vi "GD_GWID7S_info.vi"(8 "error in (no error)":errorcluster, 9 "glue_p2":sgl, 10 "glue_id":string, 11 "DBlink":string="Driver={ODBC Driver 17 for SQL Server};Server=localhost\\SQLEXPRESS;Database=ZDX201;UID=labview;PWD=Dsa@54137926") -> (0 "error out":errorcluster)   [LabVIEW 2019]
uses:
  <vilib>/addons/database/Connection.llb/DB Tools Open Connec (String).vi
  <vilib>/addons/database/NI_Database_API.lvlib
panel:
  out "Command 2":string="WHERE [id]=16"
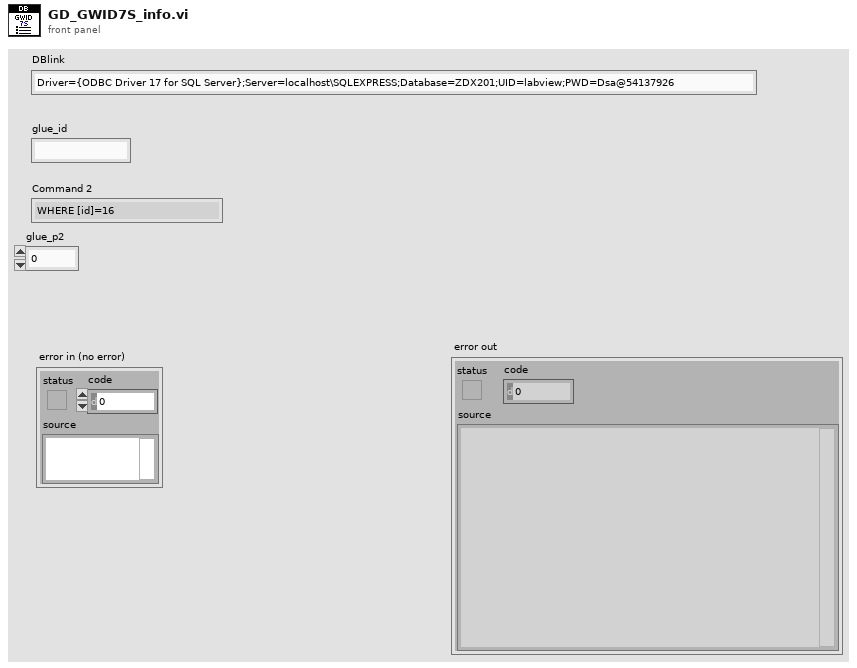
[diagram p1: front panel]
types:
  T1 = cluster{"update_time":timestamp, "time_standby_2":timestamp, "glue_p2":sgl}
  T2 = typedef "NI_Database_API.lvlib/Conn ObjectReference.ctl" = refnum<k1>
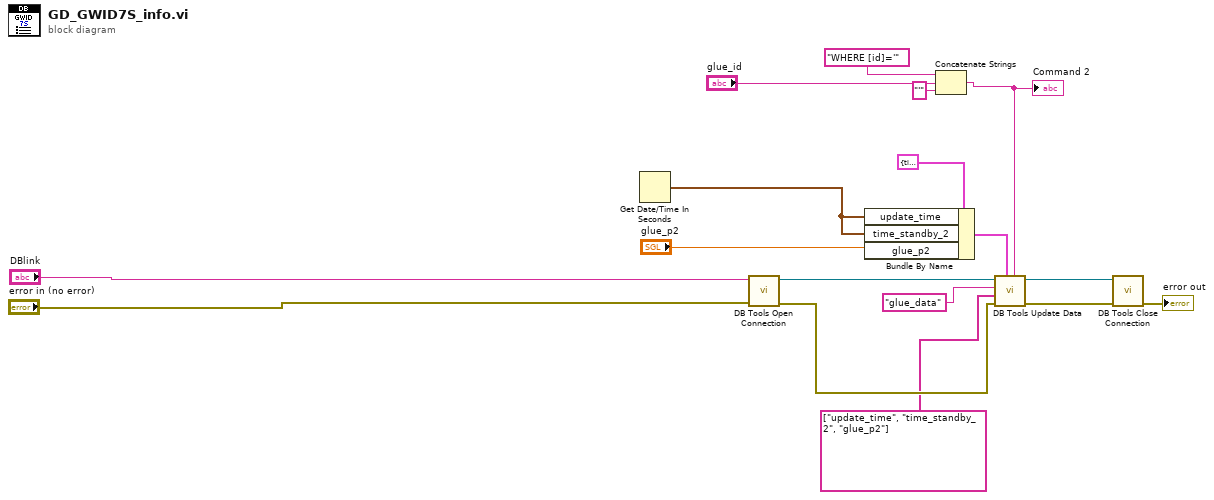
[diagram p0: block diagram]
diagram:
  n1 = Get Date/Time In Seconds() -> (seconds since 1Jan1904=w8:timestamp)
  n2 = call-poly <vilib>:"DB Tools Open Connection.vi"("error in (no error)"="error in (no error)", "connection information"="DBlink") -> ("error out"=w16:errorcluster, "connection reference"=w9:T2)  [unwired: 6 in]
  n3 = Bundle By Name(cluster=T1 {"update_time"=timestamp(0 s since 1904-01-01), "time_standby_2"=timestamp(0 s since 1904-01-01), "glue_p2"=0.0}, "update_time"=w8, "time_standby_2"=w8, "glue_p2"="glue_p2") -> (w10:T1)
  n4 = Concatenate Strings("WHERE [id]='", "glue_id", "'" ("string")) -> (w5:string)
  "Command 2" <- w5
  n5 = call <vilib>:"DB Tools Update Data.vi"("condition"=w5, "data"=w10, "error in (no error)"=w16, "columns"=string[] ["update_time", "time_standby_2", "glue_p2"], "table"="glue_data", "connection reference"=w9) -> ("error out"=w17:errorcluster, "connection reference out"=w15:T2)  [unwired: 4 in]
  n6 = call <vilib>:"DB Tools Close Connection.vi"("error in (no error)"=w17, "connection reference"=w15) -> ("error out"=→"error out":errorcluster)  [unwired: 5 in]
